vi "fmt_writeFormatBufferTails.vi"(8 "error in (no error)":errorcluster, 11 "Format buffers in":T1) -> (0 "error out":errorcluster, 3 "Format buffers out":T1)   [LabVIEW 2017, in "NI_ExcelFile.lvlib"]
uses:
  <vilib>/express/express shared/NI_ExcelFile/NI_ExcelFile.lvlib
  <vilib>/express/express shared/NI_ExcelFile/Ctrls/fmt_formatBuffer.ctl
  <vilib>/express/express shared/NI_ExcelFile/Ctrls/TimeColumnMode.ctl
  <vilib>/express/express shared/NI_ExcelFile/Ctrls/Columns.ctl
  <vilib>/express/express shared/NI_ExcelFile/Ctrls/ColumnInfo.ctl
  <vilib>/express/express shared/NI_ExcelFile/Ctrls/DataType.ctl
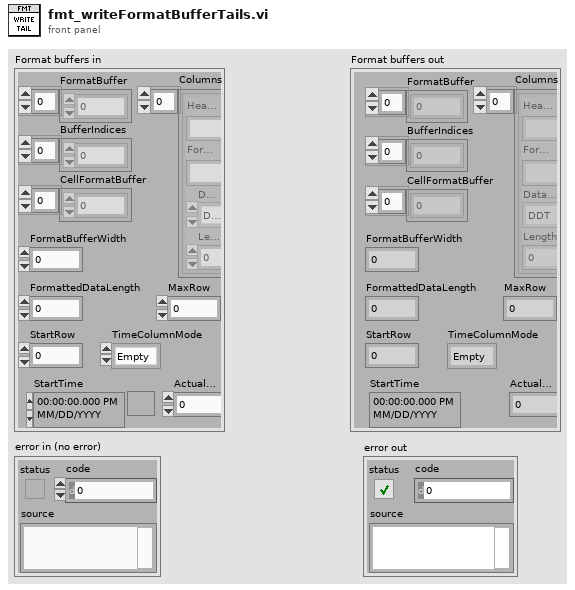
[diagram p1: front panel]
types:
  T1 = typedef "NI_ExcelFile.lvlib/fmt_formatBuffer.ctl" = cluster{"FormatBuffer":u8[], "BufferIndices":i32[], "CellFormatBuffer":u8[], "FormatBufferWidth":i32, "FormattedDataLength":i32, "MaxRow":i32, "StartRow":i32, "TimeColumnMode":T2, "StartTime":timestamp, "Columns":T3, "ActualLength":i32}
  T2 = typedef "NI_ExcelFile.lvlib/TimeColumnMode.ctl" = enum16{"Empty", "OnePerCh", "One"}
  T3 = typedef "NI_ExcelFile.lvlib/Columns.ctl" = T4[]
  T4 = typedef "NI_ExcelFile.lvlib/ColumnInfo.ctl" = cluster{"Header":string, "Format":string, "DataType":T5, "Length":u64}
  T5 = typedef "NI_ExcelFile.lvlib/DataType.ctl" = enum16{"DDT", "WFM", "Array of STR", "Array of DBL", "Array of I8", "Array of I16", "Array of I32", "Array of I64", "Array of SGL", "Array of U8", "Array of U16", "Array of U32", "Array of U64", "Array of Time"}
  T6 = typedef "LVDateTimeRec.ctl" = cluster{"fractional second":dbl, "second":i32, "minute":i32, "hour":i32, "day of month":i32, "month":i32, "year":i32, "day of week":i32, "day of year":i32, "DST":i32}
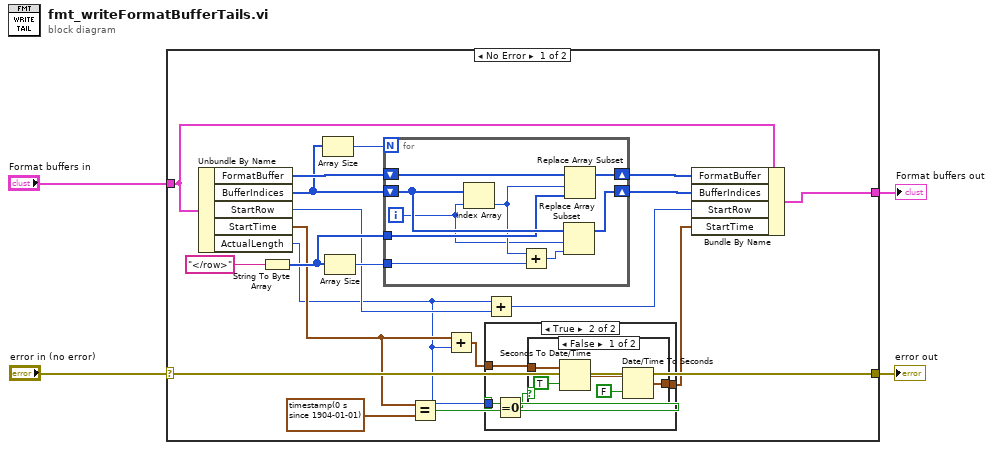
[diagram p0: block diagram]
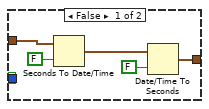
[diagram p2: hidden frame]
diagram:
  n1 = case shown="No Error" "error in (no error)" {
    selector: "error in (no error)" -> [w13 w48]
    tunnel: [w23 w49] -> w4
    tunnel: "Format buffers in" -> [w22 w49]
    tunnel: [w13 w48] -> w1
    frame No Error {
      n2 = Unbundle By Name(w22) -> ("FormatBuffer"=w21:u8[], "BufferIndices"=w17:i32[], "StartRow"=w14:i32, "StartTime"=w8:timestamp, "ActualLength"=w5:i32)
      n3 = String To Byte Array(string="</row>") -> (unsigned byte array=w16:u8[])
      n4 = Array Size(array=w17) -> (size(s)=w11:i32)
      n5 = Array Size(array=w16) -> (size(s)=w15:i32)
      n6 = for {
        N: w11 -> [_]
        shift-right: [w45] -> w19
        shift-left: w17 -> [w44]
        shift-right: [w46] -> w20
        shift-left: w21 -> [w47]
        tunnel: w16 -> [w43]
        tunnel: w15 -> [w41]
        i -> [w39]
        n7 = Index Array(array=w44, index=w39) -> (element=w42:i32)
        n8 = Add(x=w42, y=w41) -> (x+y=w40:i32)
        n9 = Replace Array Subset(array=w44, new element=w40, index=w39) -> (w45:i32[])
        n10 = Replace Array Subset(array=w47, new element=w43, index=w42) -> (w46:u8[])
      }
      n11 = Equal?(x=w8, y=timestamp(0 s since 1904-01-01)) -> (x = y?=w10:bool)
      n12 = Add(x=w8, y=w5) -> (x+y=w9:timestamp)
      n13 = case shown="True" w10 {
        tunnel: w9 -> [w28 w32]
        tunnel: [w27 w31] -> w6
        tunnel: w5 -> [_ w30]
        frame False {
          n14 = Seconds To Date/Time(time stamp (now)=w28, to UTC (F)=FALSE) -> (date time rec=w24:T6)
          n15 = Date/Time To Seconds(1:FALSE ("is UTC (F)"), 2:w24) -> (0:w27:timestamp)
        }
        frame True {
          n16 = Equal To 0?(x=w30) -> (x = 0?=w29:bool)
          n17 = case shown="False" w29 {
            tunnel: w32 -> [w34 w38]
            tunnel: [w33 w38] -> w31
            frame False {
              n18 = Seconds To Date/Time(time stamp (now)=w34, to UTC (F)=TRUE) -> (date time rec=w35:T6)
              n19 = Date/Time To Seconds(1:FALSE ("is UTC (F)"), 2:w35) -> (0:w33:timestamp)
            }
            frame True {
            }
          }
        }
      }
      n20 = Add(x=w5, y=w14) -> (x+y=w12:i32)
      n21 = Bundle By Name(cluster=w22, "FormatBuffer"=w20, "BufferIndices"=w19, "StartRow"=w12, "StartTime"=w6) -> (w23:T1)
    }
    frame Error {
    }
  }
  "Format buffers out" <- w4
  "error out" <- w1
